vi "NewTmpFile.vi"(5 "error in (no error)":errorcluster) -> (16 "path":path, 19 "error out":errorcluster)   [LabVIEW 2012, in "HGF_GPG.lvlib" / "HGF_GPG.lvclass"]
doc: "Generates Path of non-existing tmp file"
uses:
  HGF_GPG.lvclass
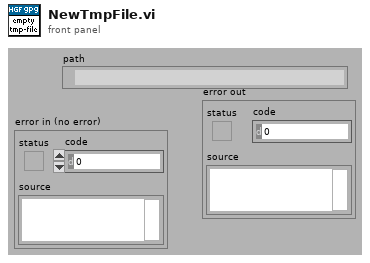
[diagram p1: front panel]
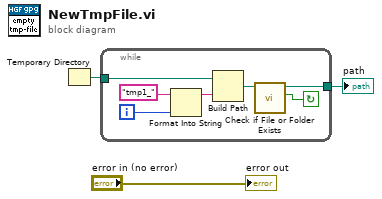
[diagram p0: block diagram]
diagram:
  n1 = Temporary Directory() -> (w2:path)
  n2 = while {
    tunnel: [w10] -> w3
    tunnel: w2 -> [w8]
    i -> [w6]
    stop <- w9 continue-if-true
    n3 = Format Into String(initial string="tmp1_" ("name or relative path"), w6) -> (resulting string=w5:string)  [unwired: 2 in, 1 out]
    n4 = Build Path(base path=w8, name or relative path=w5) -> (appended path=w4:path)
    n5 = call <vilib>:"Check if File or Folder Exists.vi"("path"=w4) -> ("file or folder exists?"=w9:bool, "dup path"=w10:path)  [unwired: 1 in, 8 out]
  }
  "path" <- w3
  "error out" <- "error in (no error)"
